vi "Get Cal Proc Docu List.vi"(6 "교정절차서 참조 배열":refnum<vi>[](array[refnum]), 8 "에러 입력(에러 없음)":errorcluster, 9 "기책 사번":string, 10 "교정정보 in":T1, 11 "참조 번호 입력":T2) -> (0 "에러 출력":errorcluster, 1 "기책 사번 out":string, 2 "교정정보 out":T1, 3 "참조 번호 출력":T2)   [LabVIEW 2020]
uses:
  <vilib>/addons/database/Connection.llb/Conn ObjectReference.ctl
  Controls/Clst_Cal Info Global.ctl
  Controls/Cmd_Read Query.ctl
  Controls/Clst_Query Info.ctl
  <vilib>/addons/database/NI_Database_API.lvlib
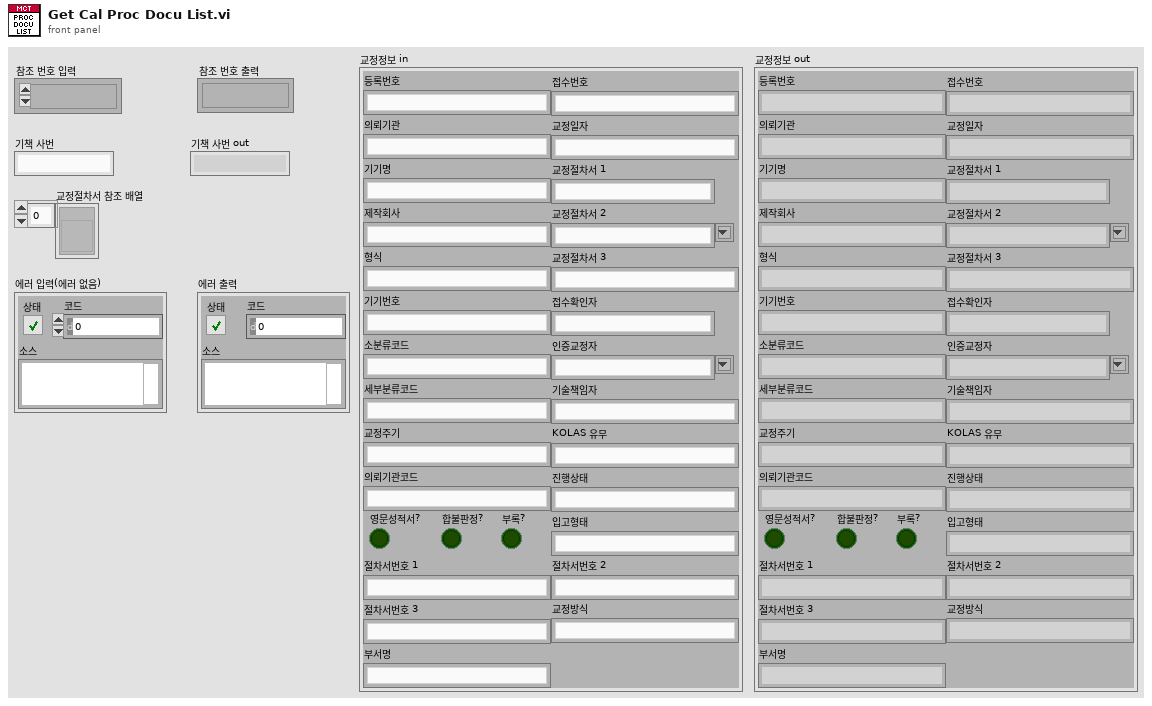
[diagram p1: front panel]
types:
  T1 = typedef "Clst_Cal Info Global.ctl" = cluster{"등록번호":string, "의뢰기관":string, "기기명":string, "제작회사":string, "형식":string, "기기번호":string, "소분류코드":string, "세부분류코드":string, "교정주기":string, "접수번호":string, "교정일자":string, "교정절차서 1":string, "교정절차서 2":string, "교정절차서 3":string, "접수확인자":string, "인증교정자":string, "기술책임자":string, "KOLAS 유무":string, "진행상태":string, "의뢰기관코드":string, "입고형태":string, "영문성적서?":bool, "합불판정?":bool, "부록?":bool, "절차서번호 1":string, "절차서번호 2":string, "절차서번호 3":string, "교정방식":string, "부서명":string}
  T2 = typedef "NI_Database_API.lvlib/Conn ObjectReference.ctl" = refnum<k1>
  T3 = typedef "Clst_Query Info.ctl" = cluster{"사번":string, "등록번호":string, "업체명":string, "세부분류코드":string, "형식":string, "기기번호":string, "FUNC":string, "FUNC_EXT":string, "옵션":string, "추가문자열":string, "일자":string, "배열 1":string[], "배열 2":string[], "항목명":string, "문자열":string, "이름":string}
  T4 = typedef "Cmd_Read Query.ctl" = enum16{"교정자 이름 얻기", "인증교정자 얻기", "기술책임자 얻기", "기책부책 얻기", "등록번호 얻기", "등록정보 얻기", "업체정보 얻기", "교정일자(CAMAS) 얻기", "교정일자(CALSTD) 얻기", "교정환경 얻기", "교정절차서 목록 얻기", "교정절차서명 얻기", "교정절차 목록얻기", "교정절차 얻기", "PROC 교정절차 얻기", "PROC SPEC 얻기", "교정절차(Func별) 얻기", "교정절차(Func_ext별) 얻기", "기관코드 얻기", "교정기능(세부분류) 얻기", "교정기능(모델) 얻기", "교정기능 목록 얻기", "교정기능 명칭 얻기", "교정기능 항목명칭 얻기", "DB (사용기준기) 얻기", "DB (기준기이름) 얻기", "DB (기준기이름목록) 얻기", "DB (기준기목록) 얻기", "DB (기준기값) 얻기", "DB (CMC) 얻기", "DB (FUNC) 얻기", "DB (CALNAME) 얻기", "DB (STDNAME) 얻기", "DB (SPEC) 얻기", "모델(항목전체) 얻기", "모델(최대범위) 얻기", "모델(최소범위) 얻기", "모델(최대최소) 얻기", "모델(범위조건) 얻기", "모델(등록요청) 얻기", "모델(형식별) 얻기", "모델(조건별) 얻기", "모델(모델검색) 얻기", "세부분류 목록 얻기", "기준기등록리스트 얻기", "STD Cal Date Check", "DB등록일자 얻기", "적용항목 얻기", "기타정보 얻기", "기준기요청 얻기", "서버버전 얻기"}
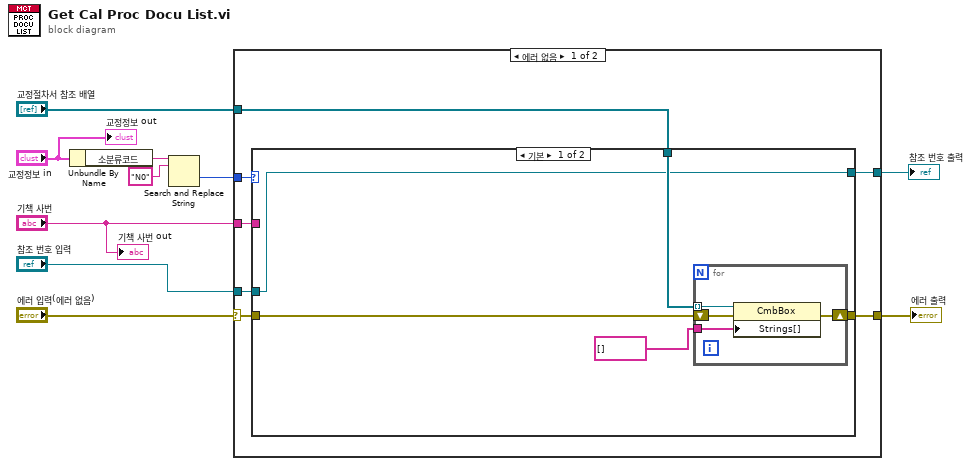
[diagram p0: block diagram]
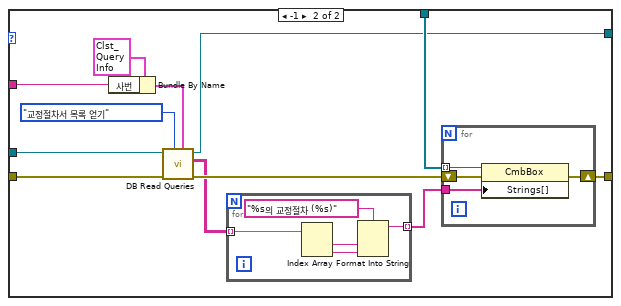
[diagram p2: hidden frame]
diagram:
  n1 = Unbundle By Name("교정정보 in") -> ("소분류코드"=w3:string)
  n2 = Search and Replace String(input string=w3, search string="N0" ("검색 문자열")) -> (offset past replacement=w1:i32)  [unwired: 6 in, 3 out]
  n3 = case shown="에러 없음" "에러 입력(에러 없음)" {
    selector: "에러 입력(에러 없음)" -> [w12 w49]
    tunnel: "교정절차서 참조 배열" -> [w17 _]
    tunnel: [w16 w49] -> w9
    tunnel: "기책 사번" -> [w15 _]
    tunnel: "참조 번호 입력" -> [w14 w48]
    tunnel: [w13 w48] -> w6
    tunnel: w1 -> [w11 _]
    frame No Error {
      n4 = case shown="기본" w11 {
        tunnel: w17 -> [w20 w37]
        tunnel: [w21 w36] -> w16
        tunnel: w15 -> [_ w33]
        tunnel: w14 -> [w19 w30]
        tunnel: [w19 w28] -> w13
        tunnel: w12 -> [w22 w27]
        frame Default {
          n5 = for {
            tunnel: w20 -> [w24] mode=indexing
            shift-right: [w25] -> w21
            shift-left: w22 -> [w26]
            tunnel: string[] [] -> [w23]
            n6 = property class="CmbBox"(reference=w24, error in=w26, "Strings[]"=w23) -> (error out=w25:errorcluster)  [unwired: 1 out]
          }
        }
        frame -1 {
          n7 = Bundle By Name(cluster=T3 {"사번"="", "등록번호"="", "업체명"="", "세부분류코드"="", "형식"="", "기기번호"="", "FUNC"="", "FUNC_EXT"="", "옵션"="", "추가문자열"="", "일자"="", "배열 1"=[], "배열 2"=[], "항목명"="", "문자열"="", "이름"=""} ("Query info"), "사번"=w33) -> (w32:T3)
          n8 = call "DB Read Queries.vi"("Query info"=w32, "Query Command"=Cmd_Read_Query."교정절차서 목록 얻기", "에러 입력(에러 없음)"=w27, "참조 번호 입력"=w30) -> ("에러 출력"=w35:errorcluster, "Data"=w34:string[][], "참조 번호 출력"=w28:T2)  [unwired: 3 in, 2 out]
          n9 = for {
            tunnel: w34 -> [w47] mode=indexing
            tunnel: [w43] -> w38 mode=indexing
            n10 = Index Array(array=w47) -> (element #1=w46:string, element #2=w45:string)  [unwired: 2 in]
            n11 = Format Into String(format string="%s의 교정절차 (%s)" ("포맷 문자열"), w46, w45) -> (resulting string=w43:string)  [unwired: 2 in, 1 out]
          }
          n12 = for {
            tunnel: w37 -> [w40] mode=indexing
            shift-right: [w41] -> w36
            shift-left: w35 -> [w42]
            tunnel: w38 -> [w39]
            n13 = property class="CmbBox"(reference=w40, error in=w42, "Strings[]"=w39) -> (error out=w41:errorcluster)  [unwired: 1 out]
          }
        }
      }
    }
    frame Error {
    }
  }
  "에러 출력" <- w9
  "참조 번호 출력" <- w6
  "기책 사번 out" <- "기책 사번"
  "교정정보 out" <- "교정정보 in"
